vi "Requests.vi"(8 "error in (no error)":errorcluster, 9 "write enable":bool=TRUE, 11 "OHAUS in":refnum<class "OHAUS_Navigator_232.lvclass">) -> (0 "error out":errorcluster, 3 "OHAUS out":refnum<class "OHAUS_Navigator_232.lvclass">)   [LabVIEW 2019, in "OHAUS_Navigator_232.lvclass"]
uses:
  OHAUS_Navigator_232.lvclass
  D:/my_projects/projects/Algorithms/Labview/19/Modbus/MB_TCP2/MB_TCP.lvclass
  OHAUS_Navigator_232.lvclass/OHAUS_Navigator_232.ctl
  Modbus/MB_TCP2/MB_TCP.lvclass/MB_TCP.ctl
  Modbus/ICPCON Registers/ICPCON Registers.lvlib
  Modbus/MB_TCP2/MB_TCP.lvclass
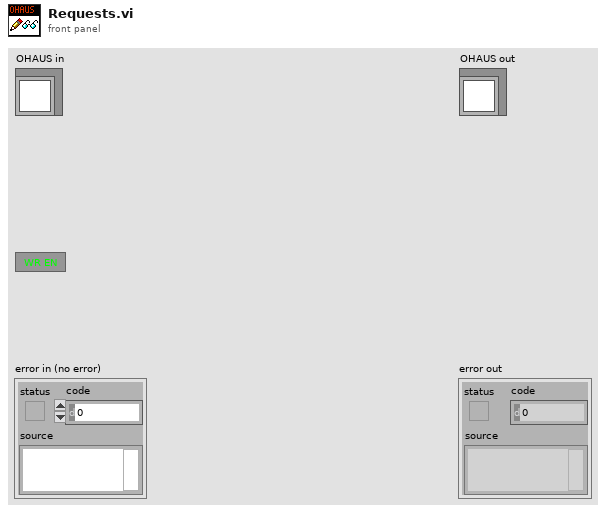
[diagram p1: front panel]
types:
  T1 = typedef "ICPCON Registers.lvlib/ICPCON Data.ctl" = cluster{"UTF":refnum<data-value>, "DI":refnum<data-value>, "DW":refnum<data-value>, "DO":refnum<data-value>, "IR":refnum<data-value>, "WR":refnum<data-value>, "OR":refnum<data-value>, "modified":refnum<data-value>}
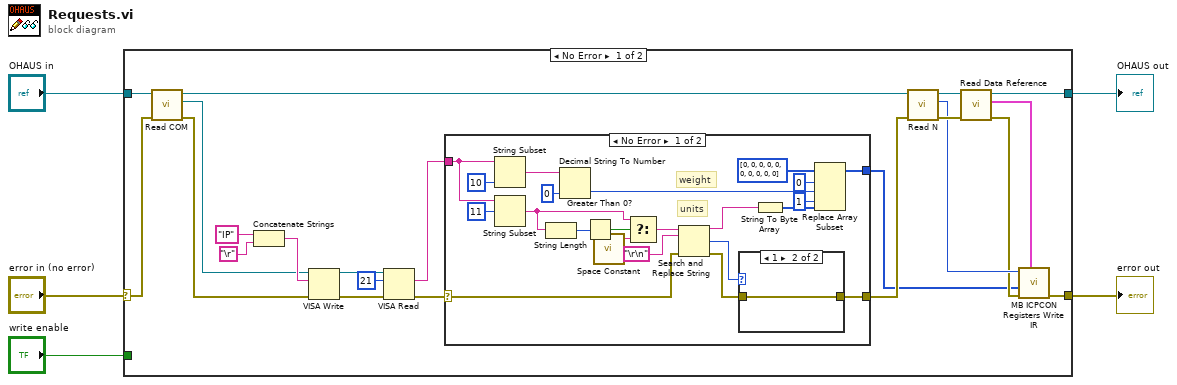
[diagram p0: block diagram]
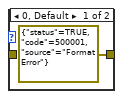
[diagram p2: hidden frame]
diagram:
  n1 = case shown="No Error" "error in (no error)" {
    selector: "error in (no error)" -> [w23 w54]
    tunnel: [w14 w54] -> w3
    tunnel: [w21 w53] -> w4
    tunnel: "OHAUS in" -> [w24 w53]
    tunnel: "write enable" -> [_ _]
    frame No Error {
      n2 = call "Read COM.vi"("error in (no error)"=w23, "OHAUS_232 in"=w24) -> ("error out"=w7:errorcluster, "COM"=w6:refnum<visa-resource-name>, "OHAUS_232 out"=w22:refnum<class "OHAUS_Navigator_232.lvclass">)  [unwired: 7 in]
      n3 = Concatenate Strings("IP" ("Code"), "\r") -> (w10:string)
      n4 = VISA Write(VISA resource name=w6, write buffer=w10, error in (no error)=w7) -> (VISA resource name out=w11:refnum<visa-resource-name>, error out=w12:errorcluster)  [unwired: 1 out]
      n5 = VISA Read(VISA resource name=w11, byte count=u32 21 ("bytes to read"), error in (no error)=w12) -> (read buffer=w9:string, error out=w8:errorcluster)  [unwired: 2 out]
      n6 = case shown="No Error" w8 {
        selector: w8 -> [w31 w52]
        tunnel: w9 -> [w45 _]
        tunnel: [w29 w52] -> w16
        tunnel: [w36 _] -> w15
        frame No Error {
          # "units"
          # "weight"
          n7 = String Subset(string=w45, length (rest)=10 ("length (rest)")) -> (substring=w47:string)  [unwired: 1 in]
          n8 = String Subset(string=w45, offset (0)=11 ("length (rest)")) -> (substring=w43:string)  [unwired: 1 in]
          n9 = String Length(string=w43) -> (length=w35:i32)
          n10 = Decimal String To Number(string=w47, default (0L)=0 ("default (0 I32)")) -> (number=w37:i32)  [unwired: 1 in, 1 out]
          n11 = Greater Than 0?(x=w35) -> (x > 0?=w44:bool)
          n12 = call <vilib>:"Space Constant.vi"() -> ("String"=w42:string)
          n13 = Select(t=w43, s=w44, f=w42) -> (s? t:f=w34:string)
          n14 = Search and Replace String(input string=w34, search string="\r\n", error in=w31) -> (result string=w33:string, number of replacements=w30:i32, error out=w28:errorcluster)  [unwired: 5 in, 1 out]
          n15 = case shown="1" w30 {
            tunnel: [errorcluster {"status"=TRUE, "code"=500001, "source"="Format Error"} ("error IO") w51] -> w29
            tunnel: w28 -> [_ w51]
            frame 0, Default {
            }
            frame 1 {
            }
          }
          n16 = String To Byte Array(string=w33) -> (unsigned byte array=w38:u8[])
          n17 = Replace Array Subset(array=u16[] [0, 0, 0, 0, 0, 0, 0, 0, 0, 0] ("Registers"), new element #1=w37, index #1=0 ("index"), new element #2=w38, index #2=1 ("index")) -> (w36:u16[])
        }
        frame Error {
        }
      }
      n18 = call "Read N.vi"("error in (no error)"=w16, "MB_TCP in"=w22) -> ("error out"=w27:errorcluster, "N"=w20:i32, "MB_TCP out"=w26:refnum<class "OHAUS_Navigator_232.lvclass">)  [unwired: 7 in]
      n19 = call "Read Data Reference.vi"("error in (no error)"=w27, "MB_TCP in"=w26) -> ("error out"=w19:errorcluster, "Data"=w25:T1, "MB_TCP out"=w21:refnum<class "OHAUS_Navigator_232.lvclass">)  [unwired: 7 in]
      n20 = call "MB ICPCON Registers Write IR.vi"("Data Reference"=w25, "error in (no error)"=w19, "Words In"=w15, "N"=w20) -> ("error out"=w14:errorcluster)  [unwired: 7 in]
    }
    frame Error {
    }
  }
  "error out" <- w3
  "OHAUS out" <- w4
